vi "EUI_6.vi"() -> ()   [LabVIEW 2018]
uses:
  <vilib>/FPGAPlugInAG/cRIO-9038/niLvFpga_Open_cRIO-9038.vi
  <vilib>/rvi/interface/common/dynamic/niFpgaDynamicAddResources.vi
  <vilib>/FPGAPlugInAG/Dynamic/niLvFpga_Run_Dynamic.vi
  <vilib>/Utility/error.llb/Error Cluster From Error Code.vi
  <vilib>/rvi/errors/niLvFpgaAdjustHostInterfaceError.vi
  <vilib>/rvi/interface/nirviOpenFPGA/nirviOpenFPGA.xnode
  Bitfiles/NiFpga_VMS_6_Controller.lvbitx
  VMS_6_Controller.vi
  <vilib>/rvi/interface/nirviMethod/nirviMethod.xnode
  <vilib>/rvi/interface/nirviReadWriteControl/nirviReadWriteControl.xnode
  <vilib>/rvi/interface/Simulation/niFpgaSimulationCallBeginRW.vi
  NiFpgaLv.dll
  <vilib>/FPGAPlugInAG/Dynamic/niLvFpga_ReadFifo_Dynamic.vi
  <vilib>/rvi/errors/niLvFpgaMergeErrorWithErrorCode.vi
panel:
  out "Numeric":i32
  out "FIFO full":bool
  out "last readout error":errorcluster
  in  "Period (ms)":i32=5
  out "error out":errorcluster
  out "Stopped":bool
  in  "Output type":T1(ring)
  out "Timeouted":bool
  out "Ticks":u64
  out "Ready":bool
  out "Accelerometers":sgl[](graph)
  in  "Operate":bool
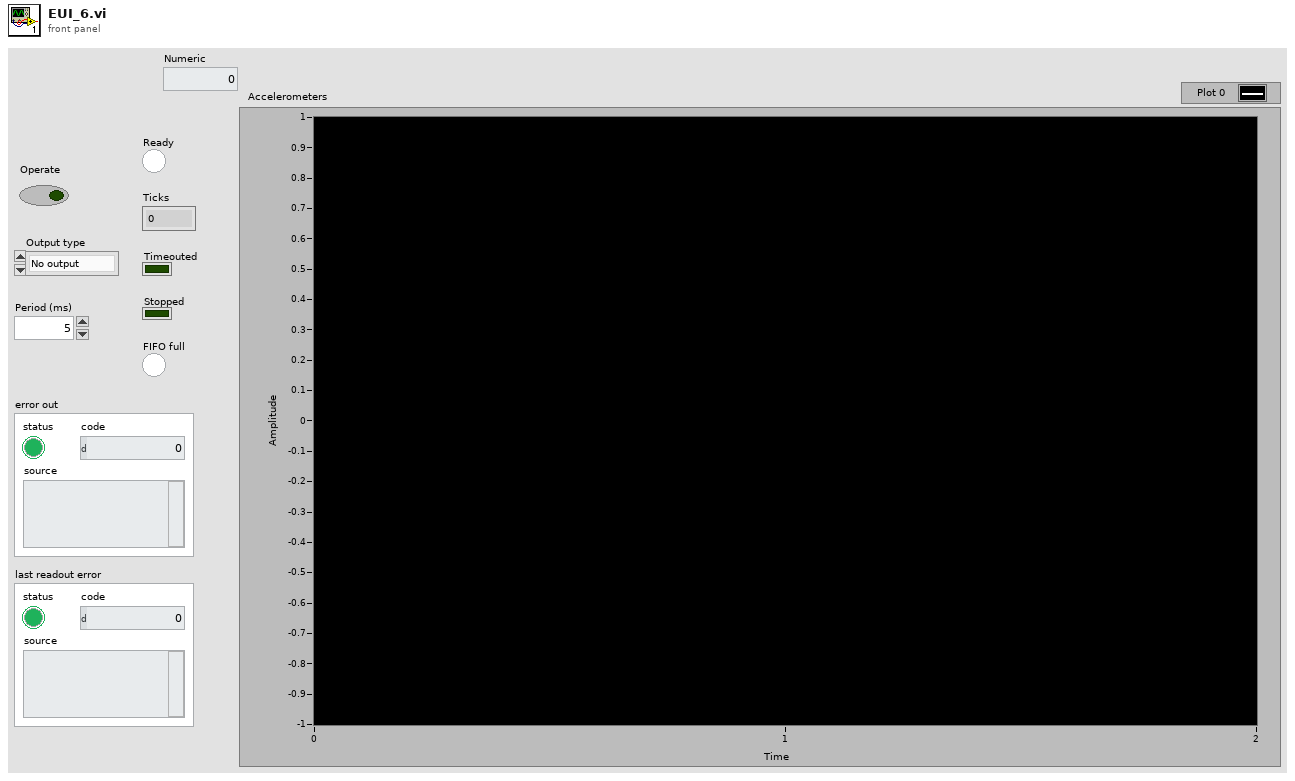
[diagram p1: front panel]
types:
  T1 = enum16{"No output", "Minimum", "Maximum", "Average"}
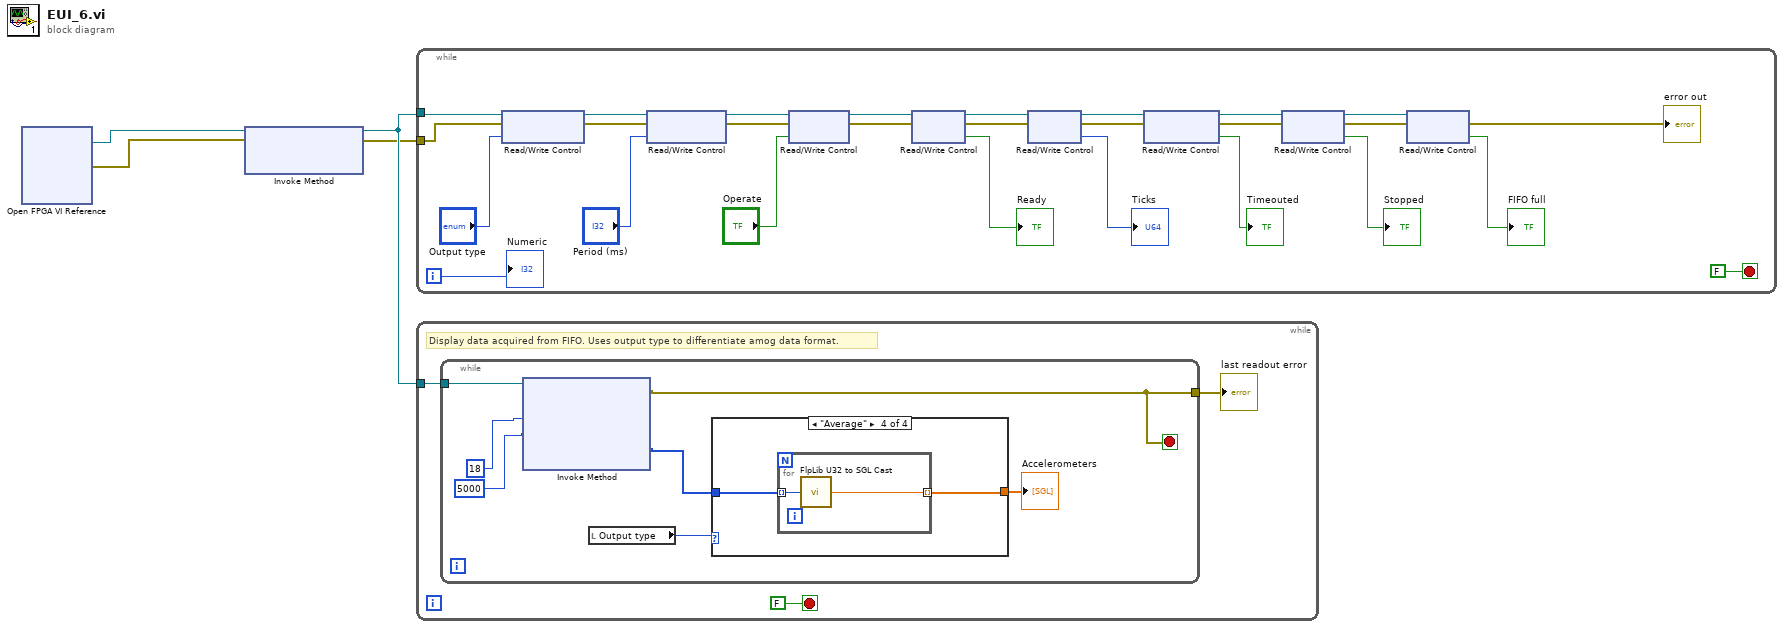
[diagram p0: block diagram]
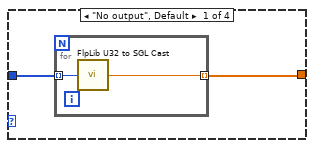
[diagram p2: hidden frame]
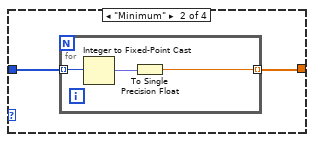
[diagram p3: hidden frame]
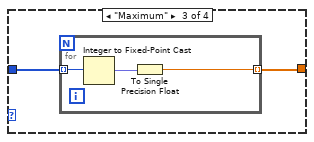
[diagram p4: hidden frame]
diagram:
  n1 = xnode "Open FPGA VI Reference"() -> ("FPGA VI Reference Out"=w1:refnum<k20>, "error out"=w2:errorcluster)  [unwired: 2 in]
  n2 = xnode "Invoke Method"("FPGA VI Reference In"=w1, "error in"=w2) -> ("FPGA VI Reference Out"=w4:refnum<k20>, "error out"=w3:errorcluster)  [unwired: 1 in]
  n3 = while {
    tunnel: w4 -> [w30]
    tunnel: w3 -> [w18]
    i -> [w5]
    stop <- FALSE stop-if-true
    n4 = xnode "Read/Write Control"("FPGA VI Reference In"=w30, "error in"=w18, "Output type"="Output type") -> ("FPGA VI Reference Out"=w22:refnum<k20>, "error out"=w12:errorcluster)
    n5 = xnode "Read/Write Control"("FPGA VI Reference In"=w22, "error in"=w12, "Period (ms)"="Period (ms)") -> ("FPGA VI Reference Out"=w13:refnum<k20>, "error out"=w11:errorcluster)
    n6 = xnode "Read/Write Control"("FPGA VI Reference In"=w13, "error in"=w11, "Operate"="Operate") -> ("FPGA VI Reference Out"=w28:refnum<k20>, "error out"=w17:errorcluster)
    n7 = xnode "Read/Write Control"("FPGA VI Reference In"=w28, "error in"=w17) -> ("FPGA VI Reference Out"=w26:refnum<k20>, "error out"=w16:errorcluster, "Ready"=→"Ready":bool)
    n8 = xnode "Read/Write Control"("FPGA VI Reference In"=w26, "error in"=w16) -> ("FPGA VI Reference Out"=w24:refnum<k20>, "error out"=w15:errorcluster, "Ticks"=→"Ticks":u64)
    n9 = xnode "Read/Write Control"("FPGA VI Reference In"=w24, "error in"=w15) -> ("FPGA VI Reference Out"=w20:refnum<k20>, "error out"=w14:errorcluster, "Timeouted"=→"Timeouted":bool)
    n10 = xnode "Read/Write Control"("FPGA VI Reference In"=w20, "error in"=w14) -> ("FPGA VI Reference Out"=w7:refnum<k20>, "error out"=w9:errorcluster, "Stopped"=→"Stopped":bool)
    n11 = xnode "Read/Write Control"("FPGA VI Reference In"=w7, "error in"=w9) -> ("error out"=→"error out":errorcluster, "FIFO full"=→"FIFO full":bool)  [unwired: 1 out]
    "Numeric" <- w5
  }
  n12 = while {
    tunnel: w4 -> [w34]
    stop <- FALSE stop-if-true
    # "Display data acquired from FIFO. Uses output type to differentiate amog data format."
    n13 = while {
      tunnel: w34 -> [w39]
      tunnel: [w38] -> w32
      stop <- w38 stop-if-true
      n14 = xnode "Invoke Method"("FPGA VI Reference In"=w39, "Number of Elements"=u32 18, "Timeout (ms)"=5000) -> ("error out"=w38:errorcluster, "Data"=w35:u32[])  [unwired: 1 in, 2 out]
      n15 = local read "Output type"() -> (w40:T1)
      n16 = case shown="\"Average\"" w40 {
        tunnel: w35 -> [w43 w47 w52 w57]
        tunnel: [w42 w46 w51 w56] -> w41
        frame "No output", Default {
          n17 = for {
            tunnel: w43 -> [w45] mode=indexing
            tunnel: [w44] -> w42 mode=indexing
            n18 = call <userlib>:"FlpLib U32 to SGL Cast.vi"("x"=w45) -> ("y"=w44:sgl)  [unwired: 4 in]
          }
        }
        frame "Minimum" {
          n19 = for {
            tunnel: w47 -> [w50] mode=indexing
            tunnel: [w48] -> w46 mode=indexing
            n20 = Integer to Fixed-Point Cast(integer=w50) -> (fixed-point=w49:fxp<+/-,24,4>)  [unwired: 1 in]
            n21 = To Single Precision Float(number=w49) -> (single precision float=w48:sgl)
          }
        }
        frame "Maximum" {
          n22 = for {
            tunnel: w52 -> [w55] mode=indexing
            tunnel: [w53] -> w51 mode=indexing
            n23 = Integer to Fixed-Point Cast(integer=w55) -> (fixed-point=w54:fxp<+/-,24,4>)  [unwired: 1 in]
            n24 = To Single Precision Float(number=w54) -> (single precision float=w53:sgl)
          }
        }
        frame "Average" {
          n25 = for {
            tunnel: w57 -> [w59] mode=indexing
            tunnel: [w58] -> w56 mode=indexing
            n26 = call <userlib>:"FlpLib U32 to SGL Cast.vi"("x"=w59) -> ("y"=w58:sgl)  [unwired: 4 in]
          }
        }
      }
      "Accelerometers" <- w41
    }
    "last readout error" <- w32
  }
